vi "IDNtest.vi"() -> ()   [LabVIEW 2013]
panel:
  out "read buffer":string
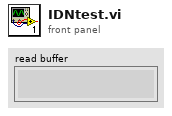
[diagram p1: front panel]
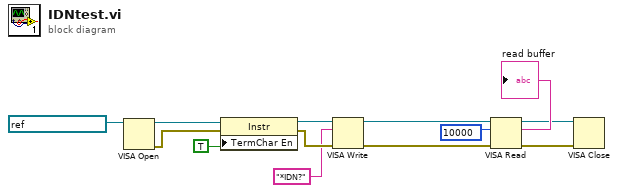
[diagram p0: block diagram]
diagram:
  n1 = VISA Open(VISA resource name=refnum<visa-resource-name> "CMW500-VXI") -> (VISA resource name=w11:refnum<visa-resource-name>, error out=w10:errorcluster)  [unwired: 4 in]
  n2 = property class="Instr"(reference=w11, error in=w10, "TermChar En"=TRUE ("Message Based Settings:Termination Character Enable")) -> (reference out=w5:refnum<visa-resource-name>, error out=w4:errorcluster)
  n3 = VISA Write(VISA resource name=w5, write buffer="*IDN?", error in (no error)=w4) -> (VISA resource name out=w7:refnum<visa-resource-name>, error out=w6:errorcluster)  [unwired: 1 out]
  n4 = VISA Read(VISA resource name=w7, byte count=u32 10000, error in (no error)=w6) -> (VISA resource name out=w2:refnum<visa-resource-name>, read buffer=→"read buffer":string, error out=w1:errorcluster)  [unwired: 1 out]
  n5 = VISA Close(VISA resource name=w2, error in (no error)=w1) -> ()  [unwired: 1 out]
